vi "Read Hardware Part Number.vi"(6 "error in":errorcluster, 8 "MaxRead":i32, 9 "Channel in":u16) -> (0 "error out":errorcluster, 1 "Messages":T1(array[cluster]) {"DATA[0]" format="%.0x"; "DATA[1]" format="%.0x"; "DATA[2]" format="%.0x"; "DATA[3]" format="%.0x"; "DATA[4]" format="%.0x"; "DATA[5]" format="%.0x"; "DATA[6]" format="%.0x"; "DATA[7]" format="%.0x"}, 2 "Pass":bool, 3 "Channel out":u16, 4 "HW Part Number":string)   [LabVIEW 2023]
uses:
  4f930f32-d09a-43ef-bca1-8b214b378bd5.vi
  e8470de1-fa2d-4ee3-b50e-96bd89dc731f.vi
  d0f02419-cfb7-4a5e-bc3c-f035efdb0e96.vi
  Communication/PCAN2023/PCAN API.lvlib
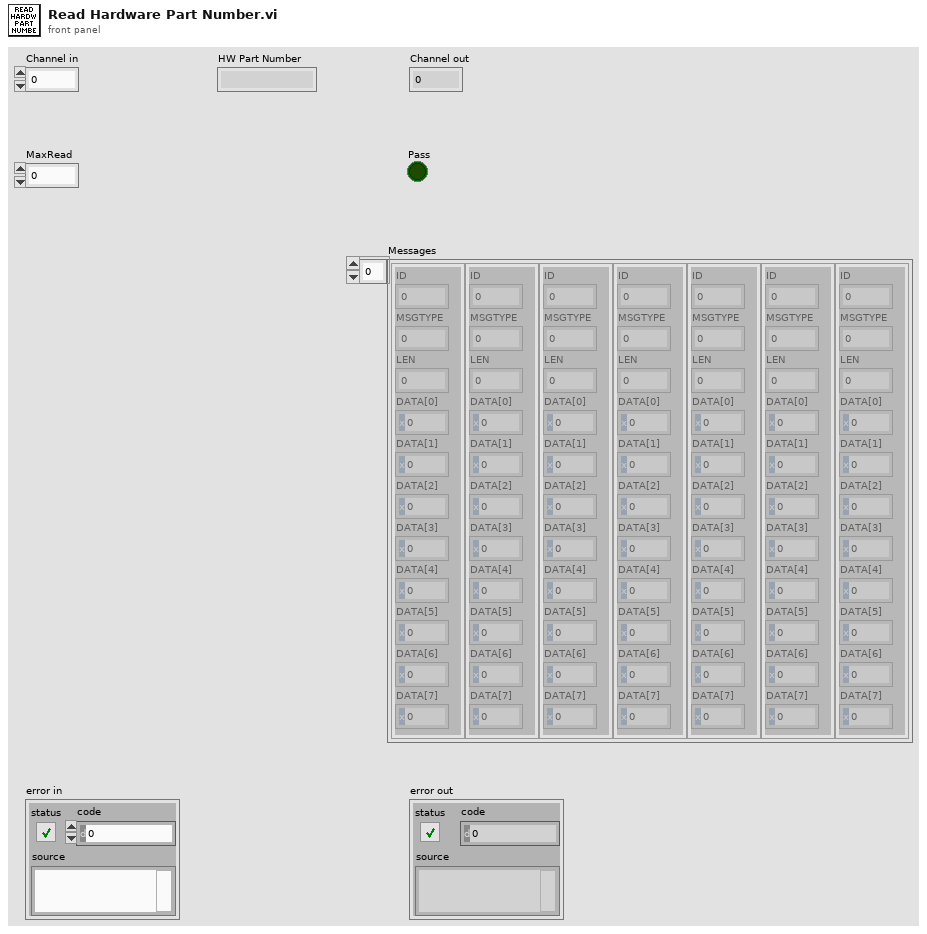
[diagram p1: front panel]
types:
  T1 = cluster{"ID":u32, "MSGTYPE":u8, "LEN":u8, "DATA[0]":u8, "DATA[1]":u8, "DATA[2]":u8, "DATA[3]":u8, "DATA[4]":u8, "DATA[5]":u8, "DATA[6]":u8, "DATA[7]":u8}[]
  T2 = cluster{"ID":u32, "MSGTYPE":u8, "LEN":u8, "DATA[0]":u8, "DATA[1]":u8, "DATA[2]":u8, "DATA[3]":u8, "DATA[4]":u8, "DATA[5]":u8, "DATA[6]":u8, "DATA[7]":u8}
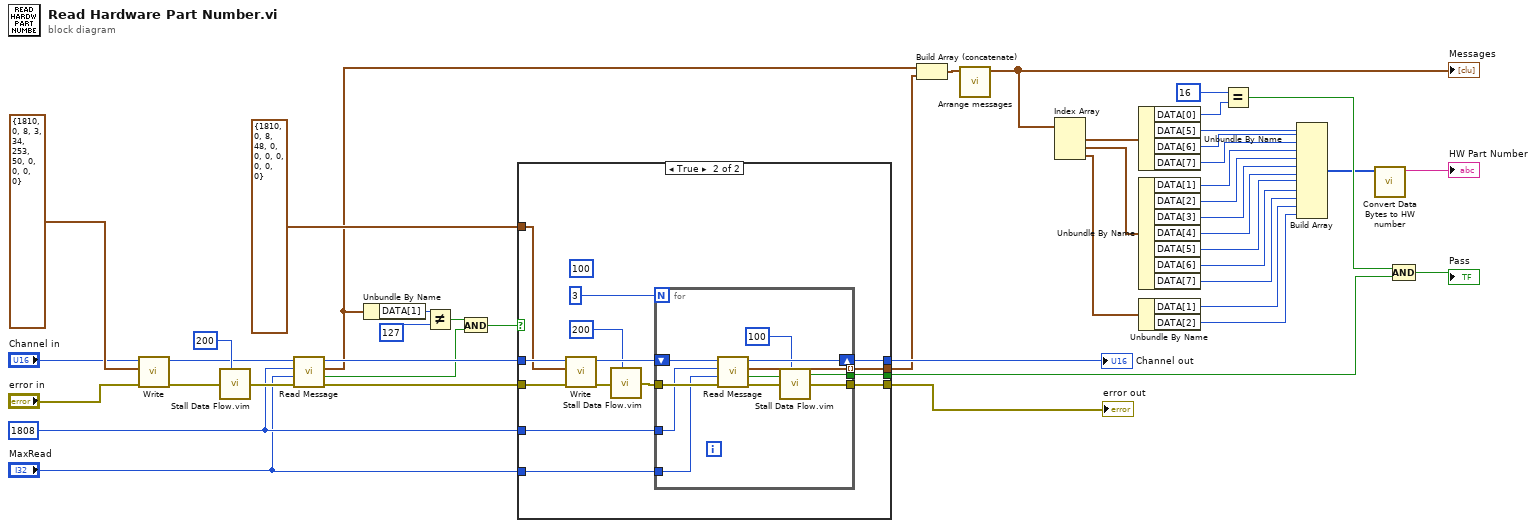
[diagram p0: block diagram]
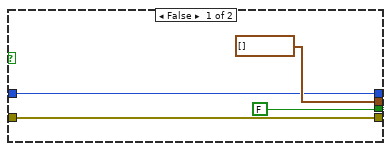
[diagram p2: hidden frame]
diagram:
  (unwired) u32 200 ("milliseconds to wait")
  w7 = u32 1808 ("ID")
  n1 = call "Write.vi"("error in"="error in", "MessageBuffer"=T2 {"ID"=1810, "MSGTYPE"=0, "LEN"=8, "DATA[0]"=3, "DATA[1]"=34, "DATA[2]"=253, "DATA[3]"=50, "DATA[4]"=0, "DATA[5]"=0, "DATA[6]"=0, "DATA[7]"=0}, "Channel"="Channel in") -> ("error out"=w40:errorcluster, "Channel out"=w15:u16)  [unwired: 5 in, 2 out]
  n2 = call "Stall Data Flow.vim"("value in"=w40, "milliseconds to wait"=u32 200) -> ("value out"=w13:errorcluster)  [unwired: 1 out]
  n3 = call "Read Message.vi"("error in"=w13, "MaxRead"="MaxRead", "ID"=w7, "Channel in"=w15) -> ("error out"=w12:errorcluster, "Passed"=w9:bool, "Last Message"=w11:T2, "Channel out"=w14:u16)  [unwired: 3 in, 1 out]
  n4 = Unbundle By Name(w11) -> ("DATA[1]"=w35:u8)
  n5 = Not Equal?(x=w35, y=u8 127) -> (x != y?=w10:bool)
  n6 = And(x=w10, y=w9) -> (x .and. y?=w8:bool)
  n7 = case shown="True" w8 {
    tunnel: w14 -> [w48 w63]
    tunnel: w12 -> [w46 w62]
    tunnel: [w46 w61] -> w39
    tunnel: [FALSE w60] -> w38
    tunnel: [w48 w58] -> w37
    tunnel: T2 {"ID"=1810, "MSGTYPE"=0, "LEN"=8, "DATA[0]"=48, "DATA[1]"=0, "DATA[2]"=0, "DATA[3]"=0, "DATA[4]"=0, "DATA[5]"=0, "DATA[6]"=0, "DATA[7]"=0} ("MessageBuffer") -> [_ w56]
    tunnel: [T1 [] w52] -> w28
    tunnel: w7 -> [_ w51]
    tunnel: "MaxRead" -> [_ w50]
    frame False {
    }
    frame True {
      (unwired) u32 100 ("milliseconds to wait")
      n8 = call "Write.vi"("error in"=w62, "MessageBuffer"=w56, "Channel"=w63) -> ("error out"=w53:errorcluster, "Channel out"=w59:u16)  [unwired: 5 in, 2 out]
      n9 = call "Stall Data Flow.vim"("value in"=w53, "milliseconds to wait"=u32 200) -> ("value out"=w57:errorcluster)  [unwired: 1 out]
      n10 = for {
        N: 3 -> [_]
        tunnel: [w65] -> w60
        shift-right: [w71] -> w58
        shift-left: w59 -> [w72]
        tunnel: w57 -> [w70]
        tunnel: [w73] -> w61
        tunnel: [w66] -> w52 mode=indexing
        tunnel: w51 -> [w68]
        tunnel: w50 -> [w67]
        n11 = call "Read Message.vi"("error in"=w70, "MaxRead"=w67, "ID"=w68, "Channel in"=w72) -> ("error out"=w69:errorcluster, "Passed"=w65:bool, "Last Message"=w66:T2, "Channel out"=w71:u16)  [unwired: 3 in, 1 out]
        n12 = call "Stall Data Flow.vim"("value in"=w69, "milliseconds to wait"=u32 100) -> ("value out"=w73:errorcluster)  [unwired: 1 out]
      }
    }
  }
  "error out" <- w39
  "Channel out" <- w37
  n13 = Build Array (concatenate)(w11, w28) -> (w5:T1)
  n14 = call "Arrange messages.vi"("Array in"=w5) -> ("Array out"=w4:T1)  [unwired: 10 in]
  "Messages" <- w4
  n15 = Index Array(array=w4) -> (element #1=w3:T2, element #2=w2:T2, element #3=w1:T2)  [unwired: 3 in]
  n16 = Unbundle By Name(w3) -> ("DATA[0]"=w26:u8, "DATA[5]"=w33:u8, "DATA[6]"=w32:u8, "DATA[7]"=w31:u8)
  n17 = Unbundle By Name(w2) -> ("DATA[1]"=w30:u8, "DATA[2]"=w25:u8, "DATA[3]"=w24:u8, "DATA[4]"=w23:u8, "DATA[5]"=w22:u8, "DATA[6]"=w21:u8, "DATA[7]"=w20:u8)
  n18 = Unbundle By Name(w1) -> ("DATA[1]"=w19:u8, "DATA[2]"=w18:u8)
  n19 = Equal?(x=u8 16 ("y"), y=w26) -> (x = y?=w29:bool)
  n20 = Build Array(w33, w32, w31, w30, w25, w24, w23, w22, w21, w20, w19, w18) -> (w17:u8[])
  n21 = call "Convert Data Bytes to HW number.vi"("Bytes"=w17) -> ("HW part number"=→"HW Part Number":string)  [unwired: 10 in]
  n22 = Compound Arithmetic op=AND(w29, w38) -> (→"Pass":bool)
